vi "Test Stub Test.vi"(8 "error in (no error)":errorcluster, 11 "LUnit Test Case.lvclass":refnum<class "LUnit Test Case.lvclass">) -> (0 "error out":errorcluster, 3 "LUnit Test Case.lvclass 2":refnum<class "LUnit Test Case.lvclass">)   [LabVIEW 2020]
uses:
  source/LUnit Test Case.lvclass
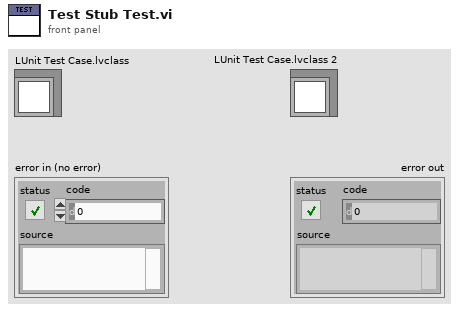
[diagram p1: front panel]
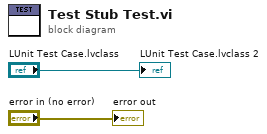
[diagram p0: block diagram]
diagram:
  "LUnit Test Case.lvclass 2" <- "LUnit Test Case.lvclass"
  "error out" <- "error in (no error)"
